vi "local VS global.vi"() -> ()   [LabVIEW 2018]
panel:
  out "LED2":bool
  out "LED 1":bool
  in  "Boolean":bool
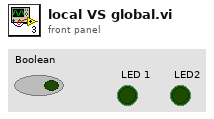
[diagram p1: front panel]
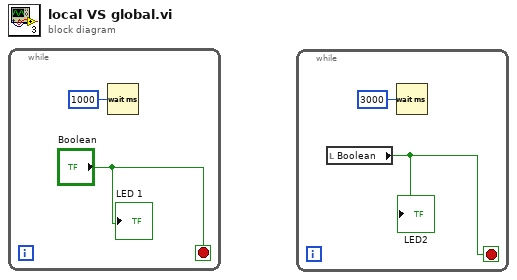
[diagram p0: block diagram]
diagram:
  n1 = while {
    stop <- "Boolean" stop-if-true
    n2 = Wait (ms)(milliseconds to wait=u32 1000) -> ()  [unwired: 1 out]
    "LED 1" <- "Boolean"
  }
  n3 = while {
    stop <- w4 stop-if-true
    n4 = local read "Boolean"() -> (w4:bool)
    "LED2" <- w4
    n5 = Wait (ms)(milliseconds to wait=u32 3000) -> ()  [unwired: 1 out]
  }
